vi "Actor Core.vi"(8 "error in":errorcluster, 11 "Camera Settings Dialog in":refnum<class "Camera Settings Dialog.lvclass">) -> (0 "error out":errorcluster, 3 "Actor out":refnum<class "Actor.lvclass">)   [LabVIEW 2014, in "Camera Settings Dialog.lvlib" / "Camera Settings Dialog.lvclass"]
doc: "(<B>Filename</B>: Actor Framework.lvlib:Actor.lvclass:Actor Core.vi)\n\nReceives messages to the actor, reacts to them, and initiates any error handling that may shut the actor down.\n\nDescendant classes may override this VI to append parallel tasks for the actor to complete while it handles messages. Overrides use the Call Parent Method node."
uses:
  Camera Settings Dialog.lvclass
  <vilib>/ActorFramework/Actor/Actor.lvclass
  Shared Code/Viewable Actor/ViewableActor/ViewableActor.lvclass/ViewableActor.ctl
  <vilib>/ActorFramework/Actor/Actor.lvclass/Actor.ctl
  <vilib>/ActorFramework/Message Enqueuer/Message Enqueuer.lvclass/Message Enqueuer.ctl
  Camera Settings Dialog.lvclass/Camera Settings Dialog.ctl
  Shared Code/Viewable Actor/ViewableActor/Write UI VI Ref.vi
  <vilib>/ActorFramework/Message Enqueuer/Init from Existing Queue.vi
  <vilib>/ActorFramework/Message Enqueuer/Enqueue.vi
  <vilib>/ActorFramework/Message Priority Queue/Priority Enqueue.vi
  <vilib>/ActorFramework/Message Enqueuer/Message Enqueuer.lvclass
  <vilib>/ActorFramework/Stop Msg/Stop Msg.lvclass
  Shared Code/Viewable Actor/ViewableActor/ViewableActor.lvclass
panel:
  in  "Stop Signal":bool=TRUE
  in  "Filter":string
  in  "Tab Control":T1(tab)
  in  "U32 Value Control":u32(slide) scale=4.0..4044.0
  in  "DBL Value Control":dbl(slide) min=17.00000029813964 max=5000000.0 step=1.0 scale=17.00000029813964..5000000.0
  in  "String Value Control":string
  in  "Enum Value Control":u32(ring) items=["Use hardware value", "10-bit", "12-bit", "14-bit", "16-bit"]
  in  "Boolean Value Control":bool=TRUE
  in  "Command Value Control":bool
  out "Tab Control Ref":T2
  in  "Attribute Table":string(tree)="_1"
  out "Units":string
  out "Tooltip":string
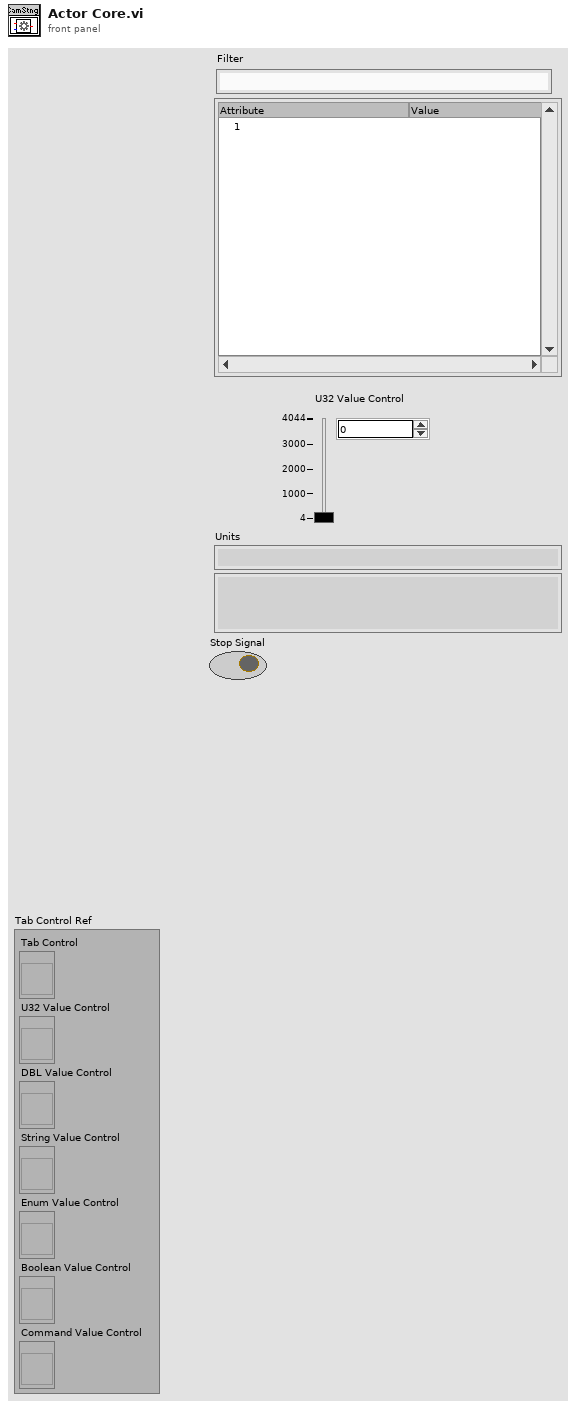
[diagram p1: front panel]
types:
  T1 = enum32{"U32", "DBL", "String", "Enum", "Bool", "Command"}
  T2 = cluster{"Tab Control":refnum<vi>, "U32 Value Control":refnum<vi>, "DBL Value Control":refnum<vi>, "String Value Control":refnum<vi>, "Enum Value Control":refnum<vi>, "Boolean Value Control":refnum<vi>, "Command Value Control":refnum<vi>}
  T3 = typedef "IMAQdx.ctl" = refnum<k21>
  T4 = typedef "eventvkey.ctl" = enum16{"ASCII", "Enter", "Return", "Shift", "Ctrl", "Alt", "Cmd", "Opt", "Caps", "NumLock", "Clear", "Break", "Up", "Down", "Left", "Right", "Insert", "Delete", "Home", "End", "PageUp", "PageDown", "Escape", "Help", "Pause", "ScrollLock", "F1", "F2", "F3", "F4", "F5", "F6", "F7", "F8", "F9", "F10", "F11", "F12", "F13", "F14", "F15", "F16", "F17", "F18", "F19", "F20", "F21", "F22", "F23", "F24", "Play", "VolumeUp", "VolumeDown", "Mute", "Two Byte Char"}
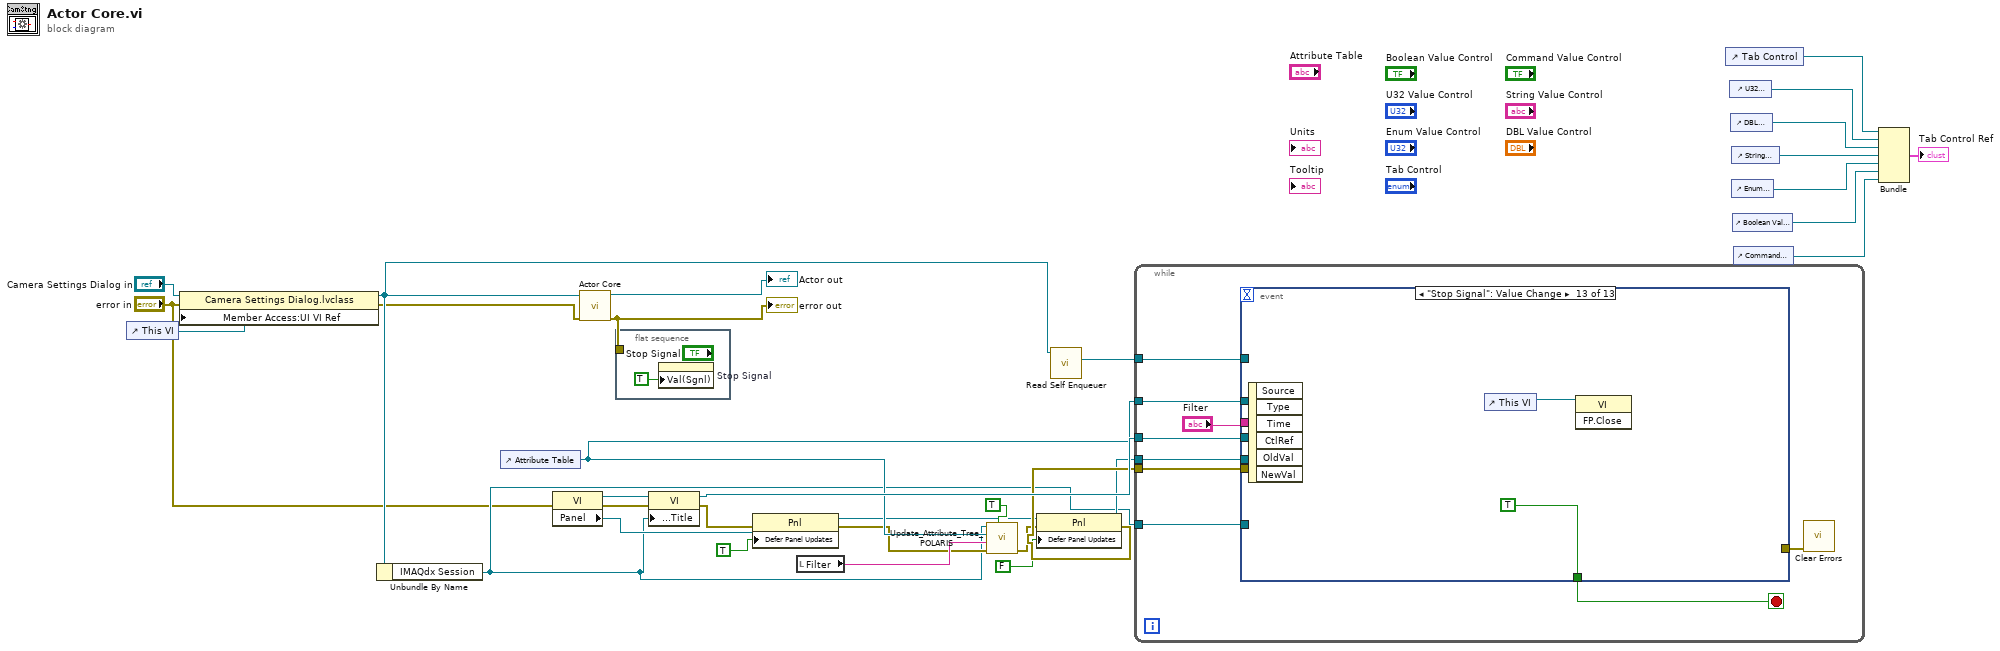
[diagram p0: block diagram]
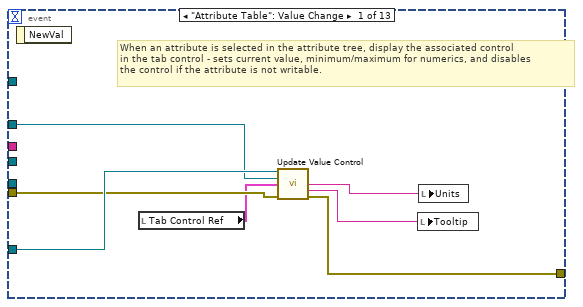
[diagram p2: hidden frame]
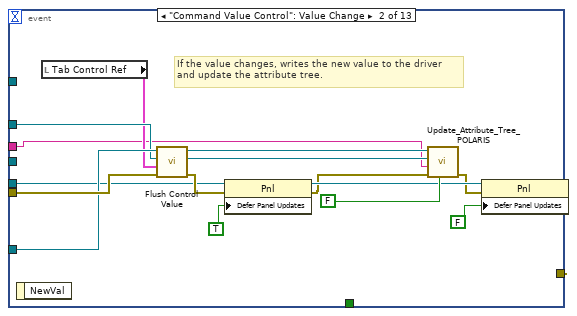
[diagram p3: hidden frame]
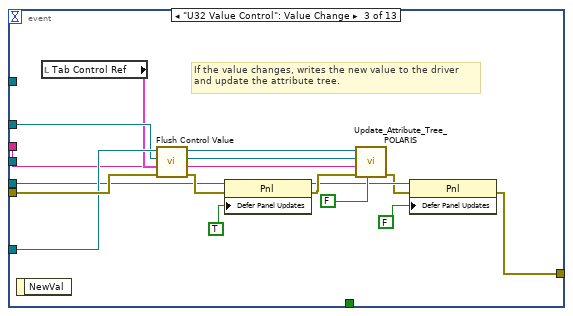
[diagram p4: hidden frame]
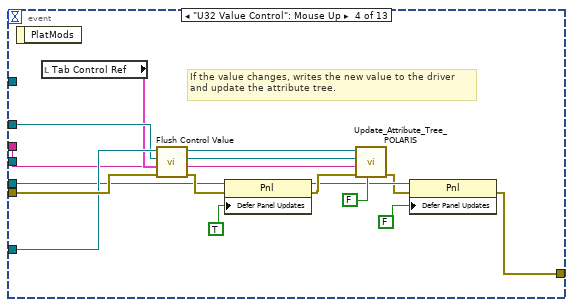
[diagram p5: hidden frame]
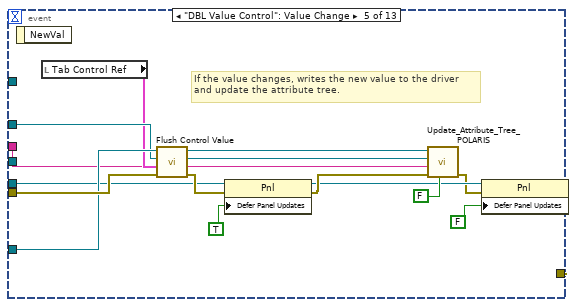
[diagram p6: hidden frame]
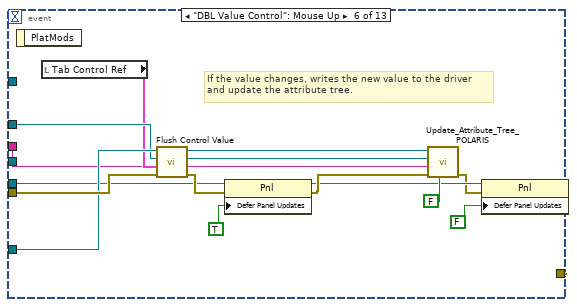
[diagram p7: hidden frame]
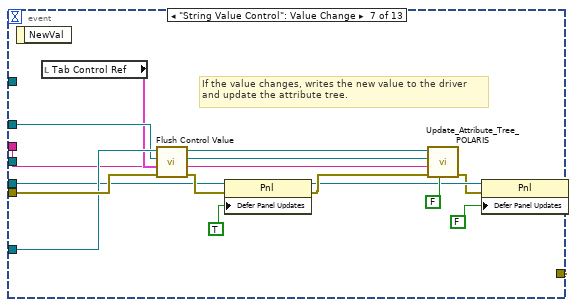
[diagram p8: hidden frame]
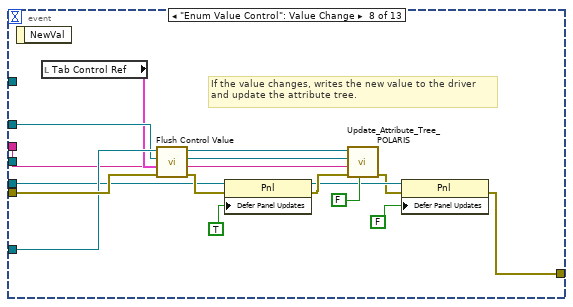
[diagram p9: hidden frame]
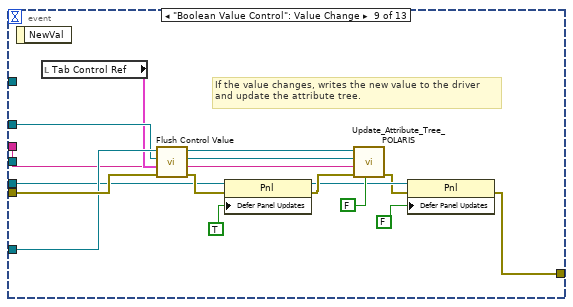
[diagram p10: hidden frame]
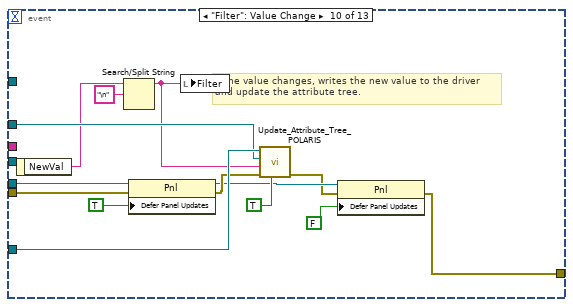
[diagram p11: hidden frame]
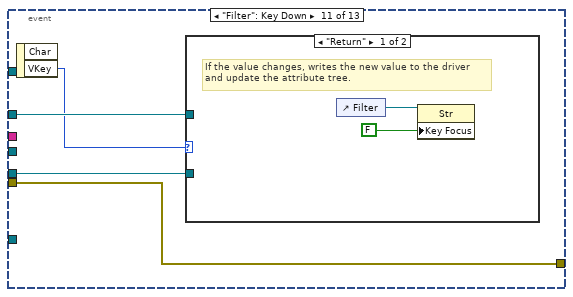
[diagram p12: hidden frame]
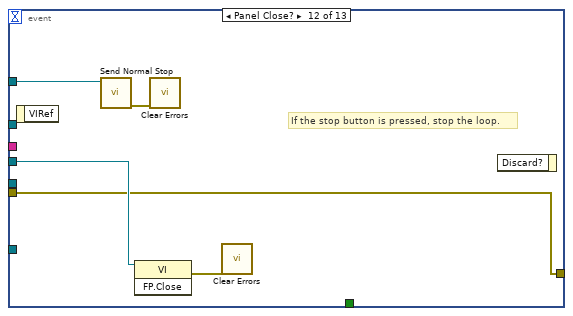
[diagram p14: hidden frame]
diagram:
  n1 = control-ref of="This VI"() -> (w3:refnum<vi>)
  n2 = property class="Camera Settings Dialog.lvclass"(reference="Camera Settings Dialog in", error in="error in", "Member Access:UI VI Ref"=w3) -> (reference out=w4:refnum<class "Camera Settings Dialog.lvclass">, error out=w1:errorcluster)
  n3 = Unbundle By Name(w4) -> ("IMAQdx Session"=w8:T3)
  n4 = control-ref of="Attribute Table"() -> (w20:refnum<vi>)
  n5 = property class="VI"(error in="error in") -> (reference out=w29:refnum<vi>, error out=w31:errorcluster, "Panel"=w27:refnum<vi>)  [unwired: 1 in]
  n6 = call-parent "Actor Core.vi"("error in"=w1, "Actor in"=w4) -> ("error out"=w7:errorcluster, "Actor out"=→"Actor out":refnum<class "Actor.lvclass">)  [unwired: 8 in]
  "error out" <- w7
  n7 = flat-sequence {
    tunnel: w7 -> [_]
    frame #0 {
      n8 = property on="Stop Signal" class="Bool (strict)"("Val(Sgnl)"=TRUE) -> ()  [unwired: 2 in, 2 out]
    }
  }
  n9 = property class="VI"(reference=w29, error in=w31, "Front Panel.Title"=w8) -> (reference out=w30:refnum<vi>, error out=w28:errorcluster)
  n10 = property class="Pnl"(reference=w27, error in=w28, "Defer Panel Updates"=TRUE) -> (reference out=w19:refnum<vi>, error out=w17:errorcluster)
  n11 = local read "Filter"() -> (w25:string)
  n12 = call "Update_Attribute_Tree_POLARIS.vi"("Flush Tree?"=TRUE, "error in"=w17, "Filter"=w25, "Tree Control In"=w20, "Camera Name In"=w8) -> ("error out"=w18:errorcluster)  [unwired: 1 in, 2 out]
  n13 = property class="Pnl"(reference=w19, error in=w18, "Defer Panel Updates"=FALSE ("Flush Tree?")) -> (reference out=w21:refnum<vi>, error out=w24:errorcluster)
  n14 = call <vilib>:"Read Self Enqueuer.vi"("Actor"=w4) -> ("Self Enqueuer"=w6:refnum<class "Message Enqueuer.lvclass">)  [unwired: 10 in]
  n15 = while {
    tunnel: w24 -> [w41]
    tunnel: w8 -> [w42]
    tunnel: w20 -> [w40]
    tunnel: w21 -> [w39]
    tunnel: w30 -> [w37]
    tunnel: w6 -> [w34]
    stop <- w38 stop-if-true
    n16 = event shown="[12] \"Stop Signal\": Value Change" {
      selector: _ -> [_ _ _ _ _ _ _ _ _ _ _ _ _]
      dyn-events: _ -> [_ _ _ _ _ _ _ _ _ _ _ _ _]
      timeout: _ -> [_ _ _ _ _ _ _ _ _ _ _ _ _]
      tunnel: w42 -> [w49 w64 w80 w96 w112 w128 w144 w160 w176 w190 _ _ _]
      tunnel: w41 -> [w48 w65 w81 w97 w113 w129 w145 w161 w177 w191 w193 w201 _]
      tunnel: [w47 w52 w67 w83 w99 w115 w131 w147 w163 w181 w193 w201 _] -> w35
      tunnel: w40 -> [w43 w62 w78 w94 w110 w126 w142 w158 w174 w189 w195 _ _]
      tunnel: w39 -> [_ w57 w72 w88 w104 w120 w136 w152 w168 w186 w194 _ _]
      tunnel: [_ _ _ _ _ _ _ _ _ _ _ _ TRUE ("stop")] -> w38
      tunnel: w37 -> [_ _ _ _ _ _ _ _ _ _ _ w202 _]
      tunnel: "Filter" -> [_ w50 w66 w82 w98 w114 w130 w146 w162 _ _ _ _]
      tunnel: w34 -> [_ _ _ _ _ _ _ _ _ _ _ w199 _]
      event "Attribute Table": Value Change {
        # "When an attribute is selected in the attribute tree, display the associated control\nin the tab control - sets current value, minimum/maximum for numerics, and disables\nthe control if the attribute is not writable."
        n17 = event-data() -> ()  [unwired: 2 out]
        n18 = local read "Tab Control Ref"() -> (w46:T2)
        n19 = call "Update Value Control.vi"("Session In"=w49, "Tree Control In"=w43, "Tab Control Ref In"=w46, "error in (no error)"=w48) -> ("Units"=w45:string, "Tooltip"=w44:string, "error out"=w47:errorcluster)  [unwired: 7 in, 2 out]
        n20 = local write "Tooltip"(w44) -> ()
        n21 = local write "Units"(w45) -> ()
      }
      event "Command Value Control": Value Change {
        # "If the value changes, writes the new value to the driver\nand update the attribute tree."
        n22 = event-data() -> ()  [unwired: 2 out]
        n23 = local read "Tab Control Ref"() -> (w61:T2)
        n24 = call "Flush Control Value.vi"("error in (no error)"=w65, "Tab Control Ref In"=w61, "Tree Control In"=w62, "Session In"=w64) -> ("error out"=w58:errorcluster, "Tree Control Out"=w60:refnum<vi>, "Session Out"=w63:T3)  [unwired: 1 in]
        n25 = property class="Pnl"(reference=w57, error in=w58, "Defer Panel Updates"=TRUE) -> (reference out=w55:refnum<vi>, error out=w51:errorcluster)
        n26 = call "Update_Attribute_Tree_POLARIS.vi"("Flush Tree?"=FALSE, "error in"=w51, "Filter"=w50, "Tree Control In"=w60, "Camera Name In"=w63) -> ("error out"=w54:errorcluster)  [unwired: 1 in, 2 out]
        n27 = property class="Pnl"(reference=w55, error in=w54, "Defer Panel Updates"=FALSE) -> (error out=w52:errorcluster)  [unwired: 1 out]
      }
      event "U32 Value Control": Value Change {
        # "If the value changes, writes the new value to the driver\nand update the attribute tree."
        n28 = event-data() -> ()  [unwired: 2 out]
        n29 = local read "Tab Control Ref"() -> (w77:T2)
        n30 = call "Flush Control Value.vi"("error in (no error)"=w81, "Tab Control Ref In"=w77, "Tree Control In"=w78, "Session In"=w80) -> ("error out"=w73:errorcluster, "Tree Control Out"=w76:refnum<vi>, "Session Out"=w79:T3)  [unwired: 1 in]
        n31 = property class="Pnl"(reference=w72, error in=w73, "Defer Panel Updates"=TRUE) -> (reference out=w70:refnum<vi>, error out=w74:errorcluster)
        n32 = call "Update_Attribute_Tree_POLARIS.vi"("Flush Tree?"=FALSE, "error in"=w74, "Filter"=w66, "Tree Control In"=w76, "Camera Name In"=w79) -> ("error out"=w69:errorcluster)  [unwired: 1 in, 2 out]
        n33 = property class="Pnl"(reference=w70, error in=w69, "Defer Panel Updates"=FALSE) -> (error out=w67:errorcluster)  [unwired: 1 out]
      }
      event "U32 Value Control": Mouse Up {
        # "If the value changes, writes the new value to the driver\nand update the attribute tree."
        n34 = event-data() -> ()  [unwired: 2 out]
        n35 = local read "Tab Control Ref"() -> (w93:T2)
        n36 = call "Flush Control Value.vi"("error in (no error)"=w97, "Tab Control Ref In"=w93, "Tree Control In"=w94, "Session In"=w96) -> ("error out"=w89:errorcluster, "Tree Control Out"=w92:refnum<vi>, "Session Out"=w95:T3)  [unwired: 1 in]
        n37 = property class="Pnl"(reference=w88, error in=w89, "Defer Panel Updates"=TRUE) -> (reference out=w86:refnum<vi>, error out=w90:errorcluster)
        n38 = call "Update_Attribute_Tree_POLARIS.vi"("Flush Tree?"=FALSE, "error in"=w90, "Filter"=w82, "Tree Control In"=w92, "Camera Name In"=w95) -> ("error out"=w85:errorcluster)  [unwired: 1 in, 2 out]
        n39 = property class="Pnl"(reference=w86, error in=w85, "Defer Panel Updates"=FALSE) -> (error out=w83:errorcluster)  [unwired: 1 out]
      }
      event "DBL Value Control": Value Change {
        # "If the value changes, writes the new value to the driver\nand update the attribute tree."
        n40 = event-data() -> ()  [unwired: 2 out]
        n41 = local read "Tab Control Ref"() -> (w109:T2)
        n42 = call "Flush Control Value.vi"("error in (no error)"=w113, "Tab Control Ref In"=w109, "Tree Control In"=w110, "Session In"=w112) -> ("error out"=w105:errorcluster, "Tree Control Out"=w108:refnum<vi>, "Session Out"=w111:T3)  [unwired: 1 in]
        n43 = property class="Pnl"(reference=w104, error in=w105, "Defer Panel Updates"=TRUE) -> (reference out=w102:refnum<vi>, error out=w106:errorcluster)
        n44 = call "Update_Attribute_Tree_POLARIS.vi"("Flush Tree?"=FALSE, "error in"=w106, "Filter"=w98, "Tree Control In"=w108, "Camera Name In"=w111) -> ("error out"=w101:errorcluster)  [unwired: 1 in, 2 out]
        n45 = property class="Pnl"(reference=w102, error in=w101, "Defer Panel Updates"=FALSE) -> (error out=w99:errorcluster)  [unwired: 1 out]
      }
      event "DBL Value Control": Mouse Up {
        # "If the value changes, writes the new value to the driver\nand update the attribute tree."
        n46 = event-data() -> ()  [unwired: 2 out]
        n47 = local read "Tab Control Ref"() -> (w125:T2)
        n48 = call "Flush Control Value.vi"("error in (no error)"=w129, "Tab Control Ref In"=w125, "Tree Control In"=w126, "Session In"=w128) -> ("error out"=w121:errorcluster, "Tree Control Out"=w124:refnum<vi>, "Session Out"=w127:T3)  [unwired: 1 in]
        n49 = property class="Pnl"(reference=w120, error in=w121, "Defer Panel Updates"=TRUE) -> (reference out=w118:refnum<vi>, error out=w122:errorcluster)
        n50 = call "Update_Attribute_Tree_POLARIS.vi"("Flush Tree?"=FALSE, "error in"=w122, "Filter"=w114, "Tree Control In"=w124, "Camera Name In"=w127) -> ("error out"=w117:errorcluster)  [unwired: 1 in, 2 out]
        n51 = property class="Pnl"(reference=w118, error in=w117, "Defer Panel Updates"=FALSE) -> (error out=w115:errorcluster)  [unwired: 1 out]
      }
      event "String Value Control": Value Change {
        # "If the value changes, writes the new value to the driver\nand update the attribute tree."
        n52 = event-data() -> ()  [unwired: 2 out]
        n53 = local read "Tab Control Ref"() -> (w141:T2)
        n54 = call "Flush Control Value.vi"("error in (no error)"=w145, "Tab Control Ref In"=w141, "Tree Control In"=w142, "Session In"=w144) -> ("error out"=w137:errorcluster, "Tree Control Out"=w140:refnum<vi>, "Session Out"=w143:T3)  [unwired: 1 in]
        n55 = property class="Pnl"(reference=w136, error in=w137, "Defer Panel Updates"=TRUE) -> (reference out=w134:refnum<vi>, error out=w138:errorcluster)
        n56 = call "Update_Attribute_Tree_POLARIS.vi"("Flush Tree?"=FALSE, "error in"=w138, "Filter"=w130, "Tree Control In"=w140, "Camera Name In"=w143) -> ("error out"=w133:errorcluster)  [unwired: 1 in, 2 out]
        n57 = property class="Pnl"(reference=w134, error in=w133, "Defer Panel Updates"=FALSE) -> (error out=w131:errorcluster)  [unwired: 1 out]
      }
      event "Enum Value Control": Value Change {
        # "If the value changes, writes the new value to the driver\nand update the attribute tree."
        n58 = event-data() -> ()  [unwired: 2 out]
        n59 = local read "Tab Control Ref"() -> (w157:T2)
        n60 = call "Flush Control Value.vi"("error in (no error)"=w161, "Tab Control Ref In"=w157, "Tree Control In"=w158, "Session In"=w160) -> ("error out"=w153:errorcluster, "Tree Control Out"=w156:refnum<vi>, "Session Out"=w159:T3)  [unwired: 1 in]
        n61 = property class="Pnl"(reference=w152, error in=w153, "Defer Panel Updates"=TRUE) -> (reference out=w150:refnum<vi>, error out=w154:errorcluster)
        n62 = call "Update_Attribute_Tree_POLARIS.vi"("Flush Tree?"=FALSE, "error in"=w154, "Filter"=w146, "Tree Control In"=w156, "Camera Name In"=w159) -> ("error out"=w149:errorcluster)  [unwired: 1 in, 2 out]
        n63 = property class="Pnl"(reference=w150, error in=w149, "Defer Panel Updates"=FALSE) -> (error out=w147:errorcluster)  [unwired: 1 out]
      }
      event "Boolean Value Control": Value Change {
        # "If the value changes, writes the new value to the driver\nand update the attribute tree."
        n64 = event-data() -> ()  [unwired: 2 out]
        n65 = local read "Tab Control Ref"() -> (w173:T2)
        n66 = call "Flush Control Value.vi"("error in (no error)"=w177, "Tab Control Ref In"=w173, "Tree Control In"=w174, "Session In"=w176) -> ("error out"=w169:errorcluster, "Tree Control Out"=w172:refnum<vi>, "Session Out"=w175:T3)  [unwired: 1 in]
        n67 = property class="Pnl"(reference=w168, error in=w169, "Defer Panel Updates"=TRUE) -> (reference out=w166:refnum<vi>, error out=w170:errorcluster)
        n68 = call "Update_Attribute_Tree_POLARIS.vi"("Flush Tree?"=FALSE, "error in"=w170, "Filter"=w162, "Tree Control In"=w172, "Camera Name In"=w175) -> ("error out"=w165:errorcluster)  [unwired: 1 in, 2 out]
        n69 = property class="Pnl"(reference=w166, error in=w165, "Defer Panel Updates"=FALSE) -> (error out=w163:errorcluster)  [unwired: 1 out]
      }
      event "Filter": Value Change {
        # "If the value changes, writes the new value to the driver\nand update the attribute tree."
        n70 = event-data() -> ("NewVal"=w180:string)  [unwired: 1 out]
        n71 = Search/Split String(string=w180, search string/char (-)="\n") -> (substring before match=w178:string)  [unwired: 1 in, 2 out]
        n72 = property class="Pnl"(reference=w186, error in=w191, "Defer Panel Updates"=TRUE) -> (reference out=w184:refnum<vi>, error out=w187:errorcluster)
        n73 = local write "Filter"(w178) -> ()
        n74 = call "Update_Attribute_Tree_POLARIS.vi"("Flush Tree?"=TRUE, "error in"=w187, "Filter"=w178, "Tree Control In"=w189, "Camera Name In"=w190) -> ("error out"=w183:errorcluster)  [unwired: 1 in, 2 out]
        n75 = property class="Pnl"(reference=w184, error in=w183, "Defer Panel Updates"=FALSE) -> (error out=w181:errorcluster)  [unwired: 1 out]
      }
      event "Filter": Key Down {
        n76 = event-data() -> ("VKey"=w192:T4)  [unwired: 2 out]
        n77 = case shown="\"Return\"" w192 {
          tunnel: w195 -> [_ _]
          tunnel: w194 -> [_ _]
          frame "Return" {
            # "If the value changes, writes the new value to the driver\nand update the attribute tree."
            n78 = control-ref of="Filter"() -> (w196:refnum<vi>)
            n79 = property class="Str"(reference=w196, "Key Focus"=FALSE) -> ()  [unwired: 1 in, 2 out]
          }
          frame "Enter", Default {
          }
        }
      }
      event Panel Close? {
        # "If the stop button is pressed, stop the loop."
        n80 = event-data() -> ()  [unwired: 2 out]
        n81 = call <vilib>:"Send Normal Stop.vi"("Message Enqueuer"=w199) -> ("error out"=w198:errorcluster)  [unwired: 10 in]
        n82 = invoke class="VI" method="FP.Close"(reference=w202) -> (error out=w200:errorcluster)  [unwired: 2 in, 2 out]
        n83 = call <vilib>:"Clear Errors.vi"("error in (no error)"=w198) -> ()  [unwired: 5 in, 2 out]
        n84 = call <vilib>:"Clear Errors.vi"("error in (no error)"=w200) -> ()  [unwired: 5 in, 2 out]
        n85 = event-data() -> ()  [unwired: 2 in, 1 out]
      }
      event "Stop Signal": Value Change {
        n86 = event-data() -> ()  [unwired: 7 out]
        n87 = control-ref of="This VI"() -> (w203:refnum<vi>)
        n88 = invoke class="VI" method="FP.Close"(reference=w203) -> ()  [unwired: 2 in, 3 out]
      }
    }
    n89 = call <vilib>:"Clear Errors.vi"("error in (no error)"=w35) -> ()  [unwired: 5 in, 2 out]
  }
  n90 = control-ref of="Tab Control"() -> (w9:refnum<vi>)
  n91 = control-ref of="U32 Value Control"() -> (w11:refnum<vi>)
  n92 = control-ref of="DBL Value Control"() -> (w12:refnum<vi>)
  n93 = control-ref of="String Value Control"() -> (w10:refnum<vi>)
  n94 = control-ref of="Enum Value Control"() -> (w13:refnum<vi>)
  n95 = control-ref of="Boolean Value Control"() -> (w14:refnum<vi>)
  n96 = control-ref of="Command Value Control"() -> (w15:refnum<vi>)
  n97 = Bundle("Tab Control"=w9, "U32 Value Control"=w11, "DBL Value Control"=w12, "String Value Control"=w10, "Enum Value Control"=w13, "Boolean Value Control"=w14, "Command Value Control"=w15) -> (→"Tab Control Ref":T2)  [unwired: 1 out]
